vi "Message_Splitter - 3 SC.vi"(10 "W2":u8[](array[numeric]), 11 "W1":u8[](array[numeric])) -> (0 "Wp2":u8[](array[numeric]), 1 "Wp1":u8[](array[numeric]), 2 "Wc2":u8[](array[numeric]), 3 "Wc1":u8[](array[numeric]))   [LabVIEW 2022 SP3]
panel:
  in  "No. Common Bits":i32=3
  in  "No. Total Bits":i32=6
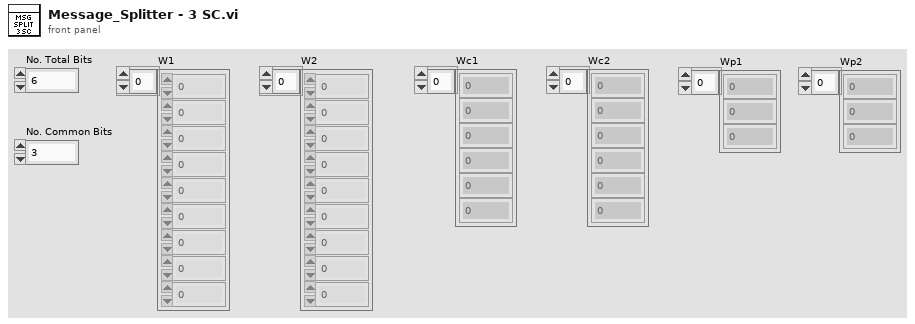
[diagram p1: front panel]
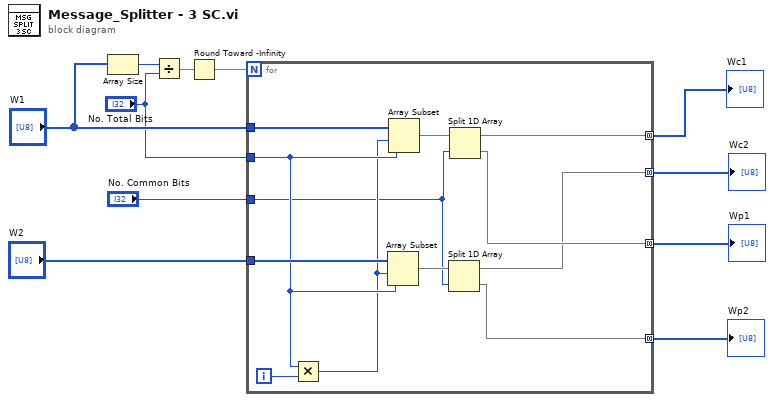
[diagram p0: block diagram]
diagram:
  n1 = Array Size(array="W1") -> (size(s)=w9:i32)
  n2 = Divide(x=w9, y="No. Total Bits") -> (x/y=w8:dbl)
  n3 = Round Toward -Infinity(1:w8) -> (0:w7:dbl)
  n4 = for {
    N: w7 -> [_]
    tunnel: "W2" -> [w22]
    tunnel: "W1" -> [w20]
    tunnel: "No. Total Bits" -> [w18]
    tunnel: [w16] -> w5 mode=concatenating
    tunnel: [w15] -> w4 mode=concatenating
    tunnel: "No. Common Bits" -> [w14]
    tunnel: [w13] -> w2 mode=concatenating
    tunnel: [w12] -> w1 mode=concatenating
    i -> [w19]
    n5 = Multiply(x=w18, y=w19) -> (x*y=w17:i32)
    n6 = Array Subset(array=w22, index=w17, length=w18) -> (w21:u8[])
    n7 = Array Subset(array=w20, index=w17, length=w18) -> (w23:u8[])
    n8 = Split 1D Array(array=w21, index=w14) -> (first subarray=w12:u8[], second subarray=w15:u8[])
    n9 = Split 1D Array(array=w23, index=w14) -> (first subarray=w13:u8[], second subarray=w16:u8[])
  }
  "Wc1" <- w2
  "Wp1" <- w5
  "Wp2" <- w4
  "Wc2" <- w1
